vi "Median Filter PtByPt.vi"(2 "initialize":bool, 3 "rank":i32=2, 5 "x":dbl format="%0.2f") -> (0 "error":i32, 1 "Filtered x":dbl format="%0.2f")   [LabVIEW 2020, in "NI_PtbyPt.lvlib"]
doc: "Applies a median filter of <B>rank</B> to <B>x</B>."
uses:
  NI_PtbyPt.lvlib
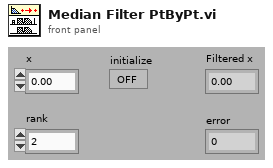
[diagram p1: front panel]
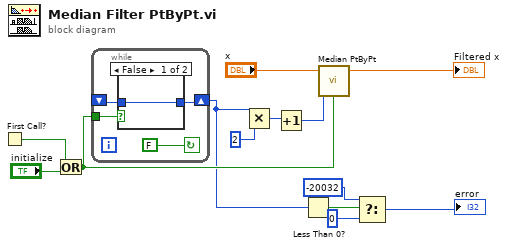
[diagram p0: block diagram]
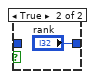
[diagram p2: hidden frame]
diagram:
  n1 = First Call?() -> (First Call?: T/F=w3:bool)
  n2 = Or(x=w3, y="initialize") -> (x .or. y?=w2:bool)
  n3 = while {
    tunnel: w2 -> [w16]
    shift-left: _ -> [w15]
    shift-right: [w17] -> w1
    stop <- FALSE continue-if-true
    n4 = case shown="False" w16 {
      tunnel: [w18 "rank"] -> w17
      tunnel: w15 -> [w18 _]
      frame False {
      }
      frame True {
      }
    }
  }
  n5 = Multiply(x=w1, y=2) -> (x*y=w12:i32)
  n6 = Increment(x=w12) -> (x+1=w11:i32)
  n7 = Less Than 0?(x=w1) -> (x < 0?=w8:bool)
  n8 = call "Median PtByPt.vi"("initialize"=w2, "sample length"=w11, "x"="x") -> ("median"=→"Filtered x":dbl)  [unwired: 1 in, 1 out]
  n9 = Select(t=-20032, s=w8, f=0) -> (s? t:f=→"error":i32)
